vi "Read Person.vi"(8 "error in (no error)":errorcluster, 11 "Person Test in":refnum<class "Person Test.lvclass">) -> (0 "error out":errorcluster, 2 "Person.lvclass":refnum<class "Person.lvclass">, 3 "Person Test out":refnum<class "Person Test.lvclass">)   [LabVIEW 2020, in "Person Test.lvclass"]
uses:
  Person Test.lvclass
  Processes/People/Person/Person.lvclass
  C:/Program Files (x86)/National Instruments/LabVIEW 2020/vi.lib/Astemes/Triarc Framework Test Suite/Base Class Test/Base Test.lvclass
  <vilib>/Astemes/Triarc Framework Test Suite/Base Class Test/Base Test.lvclass/Base Test.ctl
  <vilib>/Astemes/Triarc Framework/Base/Base.lvclass
  <vilib>/Astemes/Triarc Framework Test Suite/Base Class Test/Base Test.lvclass
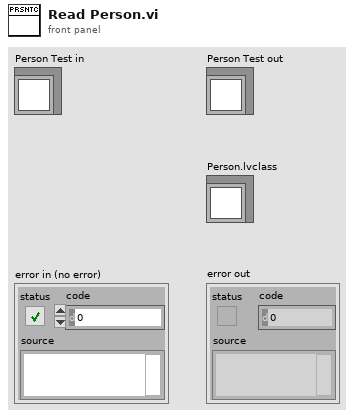
[diagram p1: front panel]
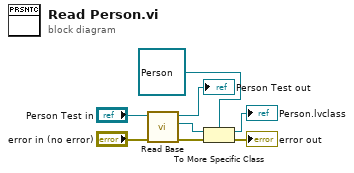
[diagram p0: block diagram]
diagram:
  n1 = call <vilib>:"Read Base.vi"("error in (no error)"="error in (no error)", "Base Class Test In"="Person Test in") -> ("error out"=w6:errorcluster, "Base.lvclass"=w5:refnum<class "Base.lvclass">, "Base Class Test Out"=→"Person Test out":refnum<class "Person Test.lvclass">)  [unwired: 7 in]
  n2 = To More Specific Class(target class=refnum<class "Person.lvclass"> refnum ("Person.lvclass"), reference=w5, error in=w6) -> (specific class reference=→"Person.lvclass":refnum<class "Person.lvclass">, error out=→"error out":errorcluster)
